vi "Read J_count.vi"(8 "error in (no error)":errorcluster, 11 "Analyze Parameter Energy per Count in":refnum<class "Analyze Parameter Energy per Count.lvclass">) -> (0 "error out":errorcluster, 2 "J/count":dbl[unit], 3 "Analyze Parameter Energy per Count out":refnum<class "Analyze Parameter Energy per Count.lvclass">)   [LabVIEW 2014, in "Analyze Parameter Energy per Count.lvclass"]
uses:
  Analyze Parameter Energy per Count.lvclass
  Analyze Parameter Energy per Count.lvclass/Analyze Parameter Energy per Count.ctl
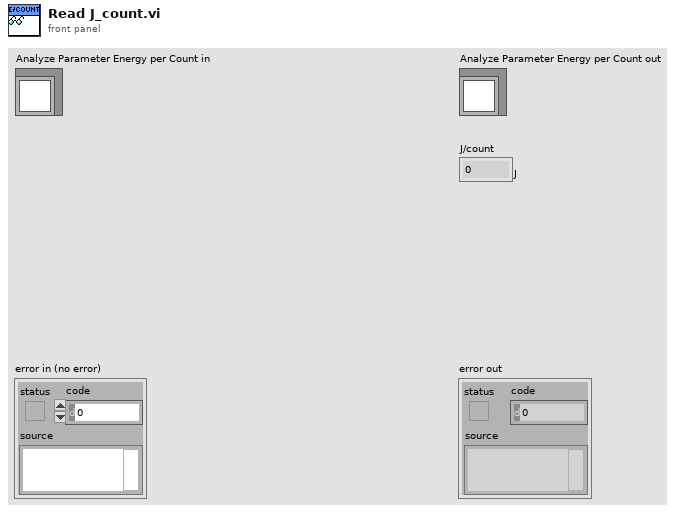
[diagram p1: front panel]
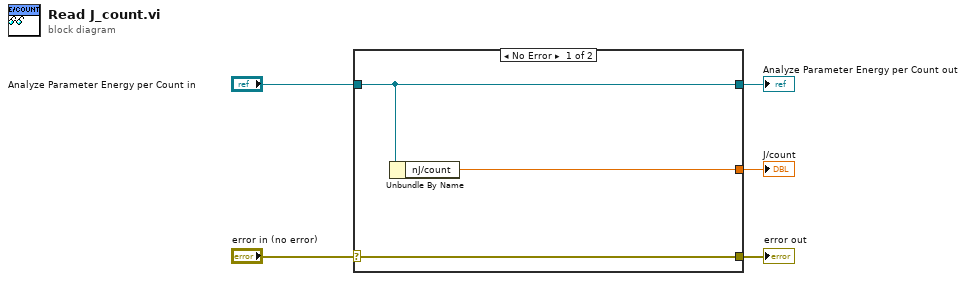
[diagram p0: block diagram]
diagram:
  n1 = case shown="No Error" "error in (no error)" {
    selector: "error in (no error)" -> [w8 w9]
    tunnel: [w8 w9] -> w4
    tunnel: [w7 w10] -> w2
    tunnel: "Analyze Parameter Energy per Count in" -> [w7 w10]
    tunnel: [w6 _] -> w1
    frame No Error {
      n2 = Unbundle By Name(w7) -> ("nJ/count"=w6:dbl[unit])
    }
    frame Error {
    }
  }
  "error out" <- w4
  "Analyze Parameter Energy per Count out" <- w2
  "J/count" <- w1
